vi "Exercise 7.2_Basic Answer.vi"() -> ()   [LabVIEW 2010]
panel:
  in  "stop":bool
  out "Locked/Unlocked":bool
  in  "Clear":bool
  out "Code Entered":string
  in  "Enter":bool
  in  "Button 9":bool
  in  "Button 8":bool
  in  "Button 7":bool
  in  "Button 6":bool
  in  "Button 5":bool
  in  "Button 4":bool
  in  "Button 3":bool
  in  "Button 2":bool
  in  "Button 1":bool
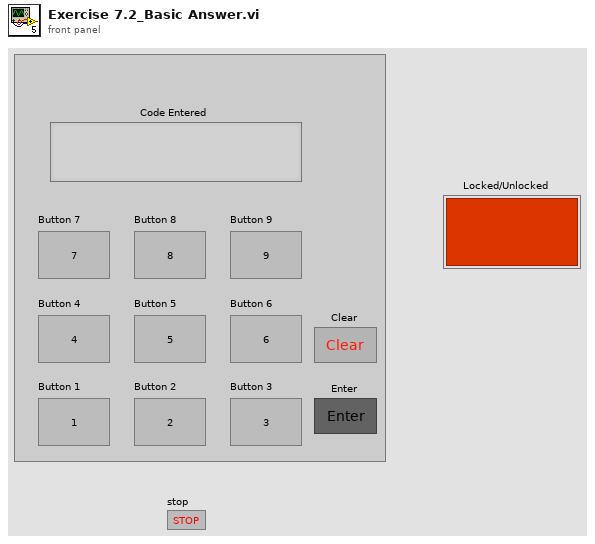
[diagram p1: front panel]
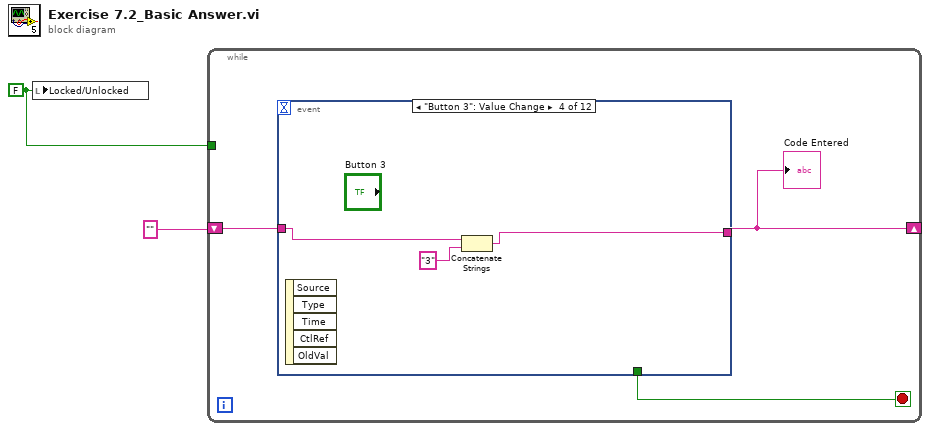
[diagram p0: block diagram]
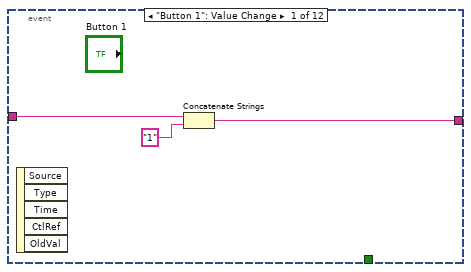
[diagram p2: hidden frame]
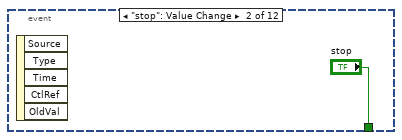
[diagram p3: hidden frame]
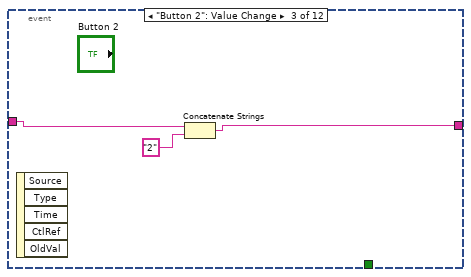
[diagram p4: hidden frame]
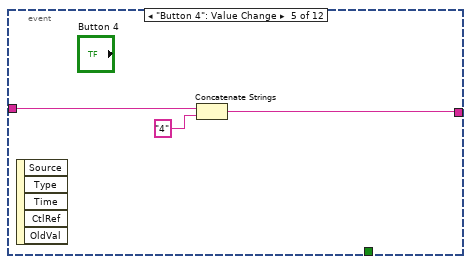
[diagram p5: hidden frame]
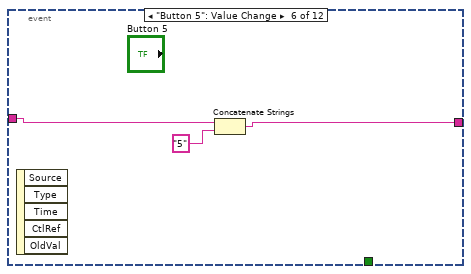
[diagram p6: hidden frame]
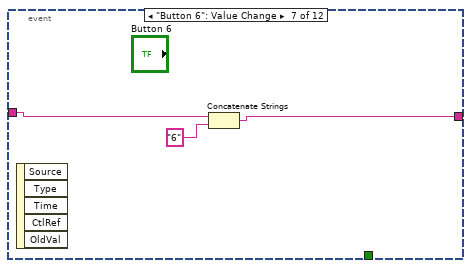
[diagram p7: hidden frame]
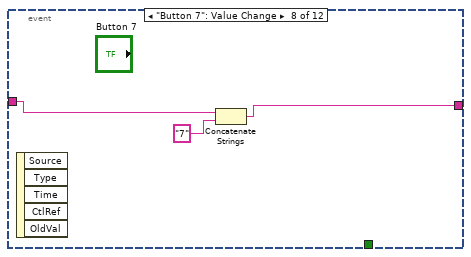
[diagram p8: hidden frame]
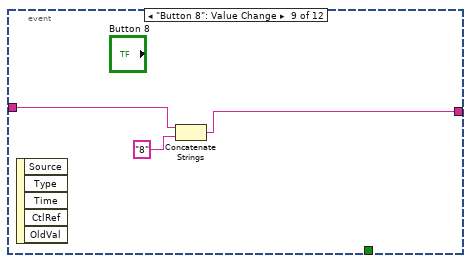
[diagram p9: hidden frame]
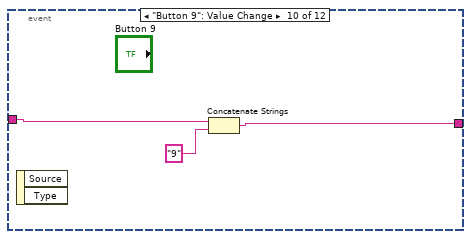
[diagram p10: hidden frame]
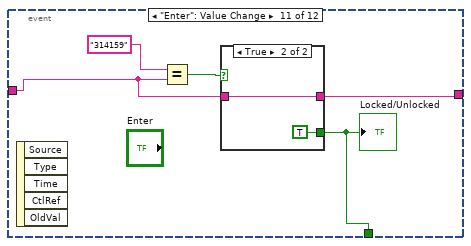
[diagram p11: hidden frame]
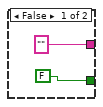
[diagram p12: hidden frame]
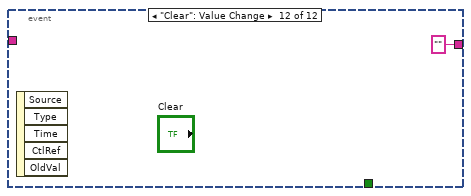
[diagram p13: hidden frame]
diagram:
  w1 = FALSE ("Locked/Unlocked")
  n1 = local write "Locked/Unlocked"(w1) -> ()
  n2 = while {
    shift-right: [w4] -> _
    shift-left: "" -> [w5]
    tunnel: w1 -> [_]
    stop <- w3 stop-if-true
    n3 = event shown="[3] \"Button 3\": Value Change" {
      selector: _ -> [_ _ _ _ _ _ _ _ _ _ _ _]
      dyn-events: _ -> [_ _ _ _ _ _ _ _ _ _ _ _]
      timeout: _ -> [_ _ _ _ _ _ _ _ _ _ _ _]
      tunnel: w5 -> [w8 _ w11 w14 w17 w20 w23 w26 w29 w32 w36 _]
      tunnel: [w6 _ w10 w13 w16 w19 w22 w25 w28 w31 w35 ""] -> w4
      tunnel: [_ "stop" _ _ _ _ _ _ _ _ w34 _] -> w3
      event "Button 1": Value Change {
        n4 = event-data() -> ()  [unwired: 1 in, 5 out]
        n5 = Concatenate Strings(w8, "1" ("string")) -> (w6:string)
      }
      event "stop": Value Change {
        n6 = event-data() -> ()  [unwired: 1 in, 5 out]
      }
      event "Button 2": Value Change {
        n7 = event-data() -> ()  [unwired: 1 in, 5 out]
        n8 = Concatenate Strings(w11, "2" ("string")) -> (w10:string)
      }
      event "Button 3": Value Change {
        n9 = event-data() -> ()  [unwired: 1 in, 5 out]
        n10 = Concatenate Strings(w14, "3" ("string")) -> (w13:string)
      }
      event "Button 4": Value Change {
        n11 = event-data() -> ()  [unwired: 1 in, 5 out]
        n12 = Concatenate Strings(w17, "4" ("string")) -> (w16:string)
      }
      event "Button 5": Value Change {
        n13 = event-data() -> ()  [unwired: 1 in, 5 out]
        n14 = Concatenate Strings(w20, "5" ("string")) -> (w19:string)
      }
      event "Button 6": Value Change {
        n15 = event-data() -> ()  [unwired: 1 in, 5 out]
        n16 = Concatenate Strings(w23, "6" ("string")) -> (w22:string)
      }
      event "Button 7": Value Change {
        n17 = event-data() -> ()  [unwired: 1 in, 5 out]
        n18 = Concatenate Strings(w26, "7" ("string")) -> (w25:string)
      }
      event "Button 8": Value Change {
        n19 = event-data() -> ()  [unwired: 1 in, 5 out]
        n20 = Concatenate Strings(w29, "8" ("string")) -> (w28:string)
      }
      event "Button 9": Value Change {
        n21 = event-data() -> ()  [unwired: 1 in, 2 out]
        n22 = Concatenate Strings "Concatenate Strings"(w32, "9" ("string")) -> (w31:string)
      }
      event "Enter": Value Change {
        n23 = event-data() -> ()  [unwired: 1 in, 5 out]
        n24 = Equal?(x="314159", y=w36) -> (x = y?=w37:bool)
        n25 = case shown="True" w37 {
          tunnel: w36 -> [_ w42]
          tunnel: ["" w42] -> w35
          tunnel: [FALSE ("Locked/Unlocked") TRUE ("Locked/Unlocked")] -> w34
          frame False {
          }
          frame True {
          }
        }
        "Locked/Unlocked" <- w34
      }
      event "Clear": Value Change {
        n26 = event-data() -> ()  [unwired: 1 in, 5 out]
      }
    }
    "Code Entered" <- w4
  }
